vi "Write Array.vi"(8 "Error In":errorcluster, 10 "Name":string, 11 "Variant":variant) -> (0 "Error Out":errorcluster, 3 "String":string)   [LabVIEW 2017, in "Configit.lvlib"]
uses:
  Configit.lvlib
  <vilib>/Utility/VariantDataType/Type.ctl
  <vilib>/Waveform/DWDTOps.llb/DWDT Empty Digital.vi
  <vilib>/Waveform/DTblOps.llb/DTbl Empty Digital.vi
  <vilib>/Utility/VariantDataType/VariantType.lvlib
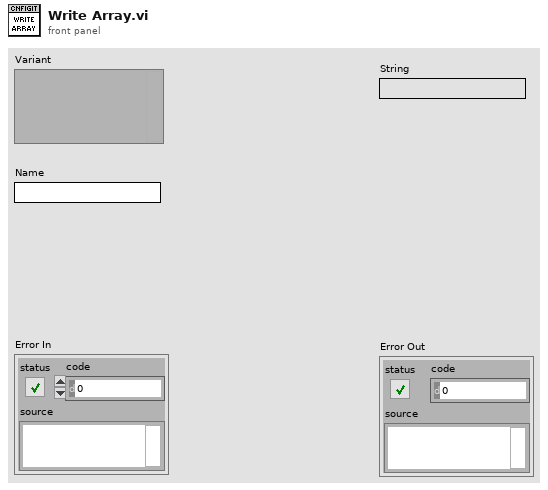
[diagram p1: front panel]
types:
  T1 = typedef "VariantType.lvlib/Type.ctl" = enum8{"Invalid Type", "Void", "I8", "I16", "I32", "I64", "U8", "U16", "U32", "U64", "Single Float", "Double Float", "Extended Float", "Single Complex", "Double Complex", "Extended Complex", "Enum U8", "Enum U16", "Enum U32", "Enum U64", "Single Float With Unit", "Double Float With Unit", "Extended Float With Unit", "Single Complex with Unit", "Double Complex with Unit", "Extended Complex with Unit", "Boolean", "String", "Path", "Picture", "Tag", "Array", "Cluster", "Variant", "LV Variant", "Waveform", "Timestamp", "Digital Waveform", "Digital Data", "ExpressData", "Refnum", "External Data", "VI", "Poly VI", "LabVIEW Class Instance", "Fixed Point"}
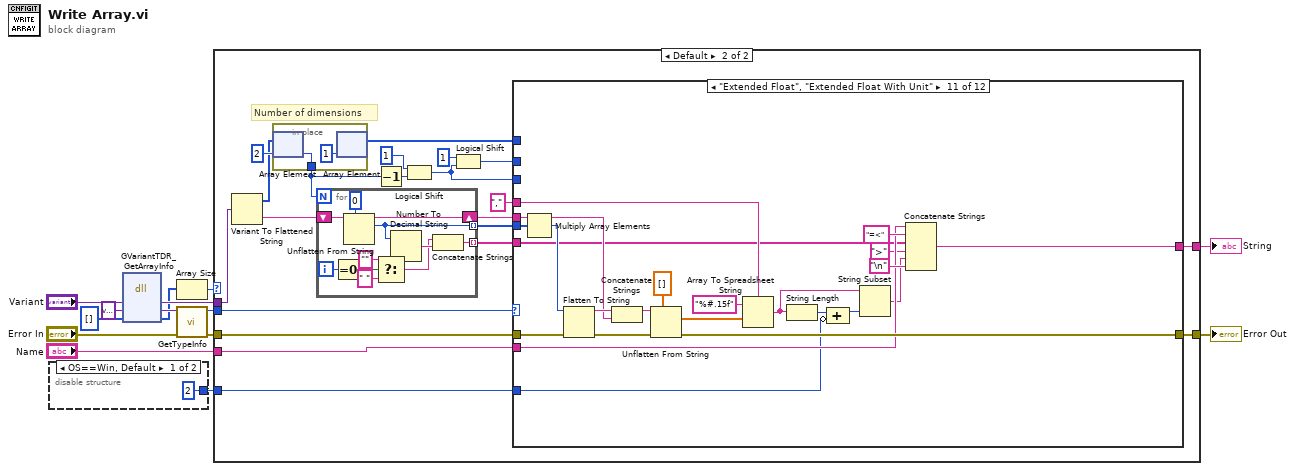
[diagram p0: block diagram]
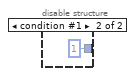
[diagram p2: hidden frame]
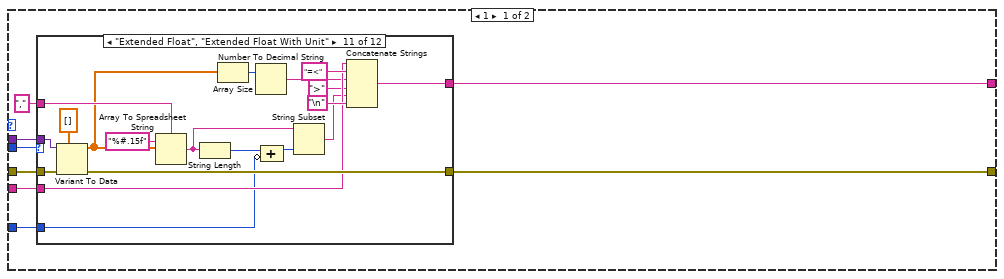
[diagram p3: hidden frame]
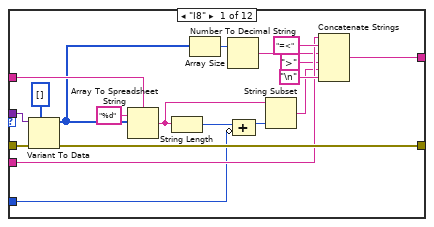
[diagram p4: hidden frame]
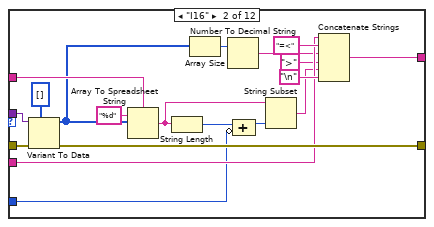
[diagram p5: hidden frame]
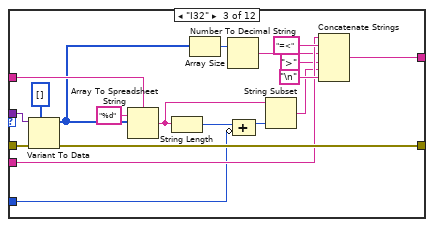
[diagram p6: hidden frame]
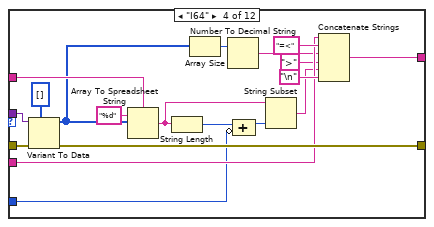
[diagram p7: hidden frame]
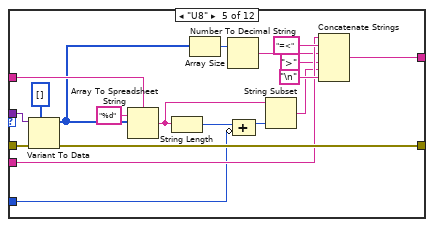
[diagram p8: hidden frame]
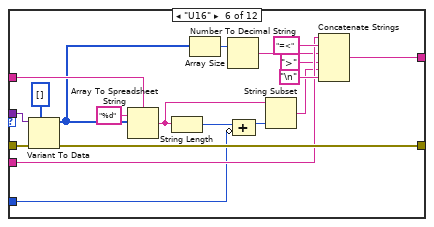
[diagram p9: hidden frame]
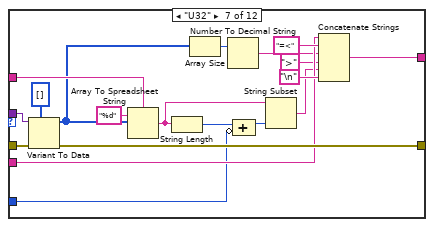
[diagram p10: hidden frame]
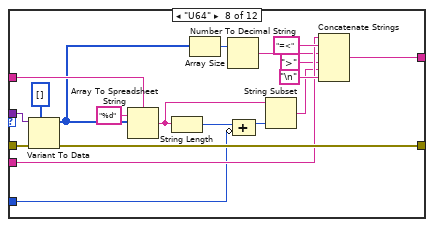
[diagram p11: hidden frame]
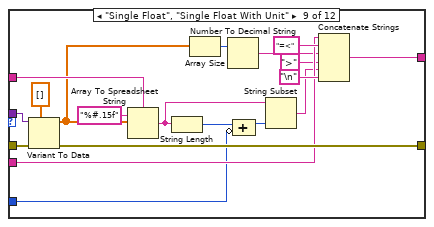
[diagram p12: hidden frame]
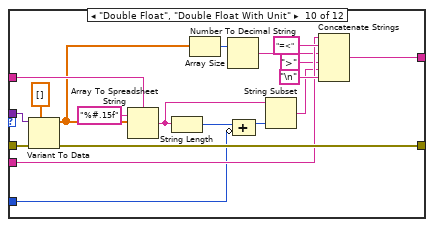
[diagram p13: hidden frame]
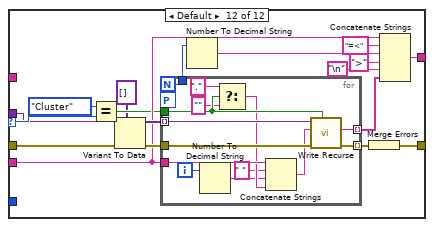
[diagram p14: hidden frame]
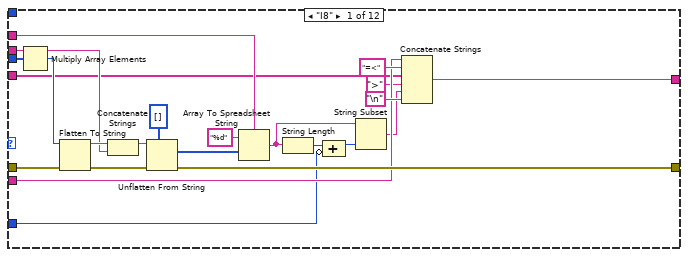
[diagram p15: hidden frame]
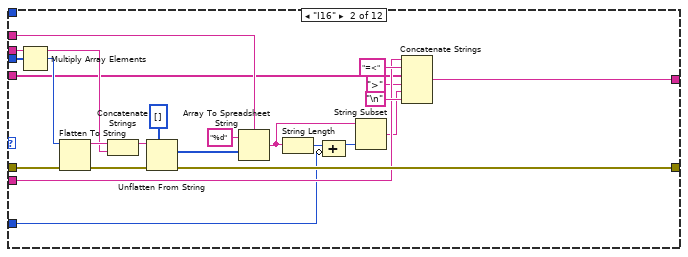
[diagram p16: hidden frame]
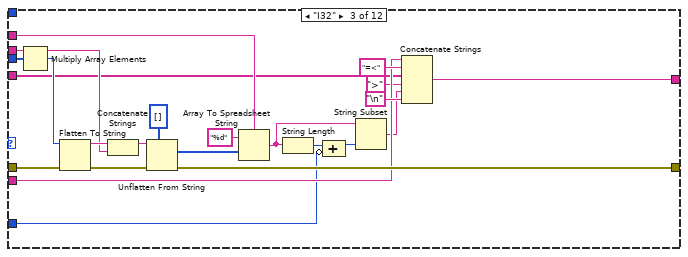
[diagram p17: hidden frame]
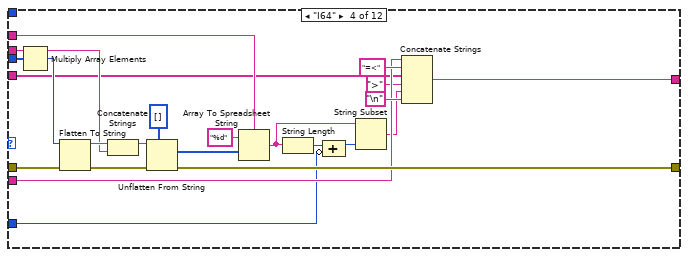
[diagram p18: hidden frame]
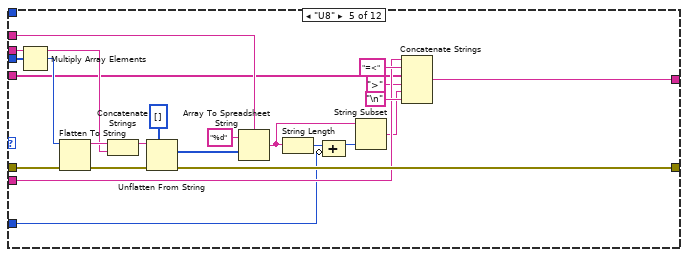
[diagram p19: hidden frame]
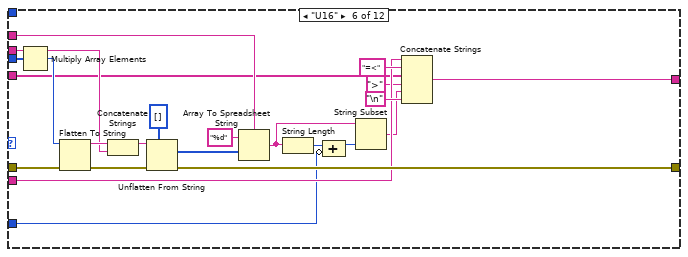
[diagram p20: hidden frame]
diagram:
  n1 = disable-structure shown="OS==Win, Default" {
    disable-tunnel: [2 ("value") 1 ("value")] -> w1
    frame condition #0 (active) {
    }
    frame condition #1 {
    }
  }
  n2 = dll-call lib="LabVIEW" fn="GVariantTDR_GetArrayInfo"("lvVar"="Variant", "eltType"=variant ("ArrayElt"), "dimInfo"=i32[] []) -> ("lvVar"=w4:variant, "eltType"=w6:variant, "dimInfo"=w3:i32[])  [unwired: 4 in, 2 out]
  n3 = Array Size(array=w3) -> (size(s)=w2:i32)
  n4 = call "GetTypeInfo.vi"("Error In"="Error In", "Variant"=w6) -> ("Error Out"=w13:errorcluster, "Type Enum"=w14:T1)  [unwired: 6 in, 2 out]
  n5 = case shown="Default" w2 {
    tunnel: w14 -> [w24 w284]
    tunnel: w13 -> [w23 w283]
    tunnel: [w21 w279] -> w12
    tunnel: [w20 w278] -> w11
    tunnel: "Name" -> [w19 w277]
    tunnel: w4 -> [w18 w276]
    tunnel: w1 -> [w17 w266]
    frame 1 {
      n6 = case shown="\"Extended Float\", \"Extended Float With Unit\"" w24 {
        selector: w24 -> [_ _ _ _ _ _ _ _ _ _ _ w246]
        tunnel: w23 -> [w34 w53 w72 w91 w110 w129 w148 w167 w186 w205 w224 w237]
        tunnel: "," -> [w41 w60 w79 w98 w117 w136 w155 w174 w193 w212 w231 _]
        tunnel: [w38 w57 w76 w95 w114 w133 w152 w171 w190 w209 w228 w248] -> w21
        tunnel: [w37 w56 w75 w94 w113 w132 w151 w170 w189 w208 w227 w247] -> w20
        tunnel: w19 -> [w36 w55 w74 w93 w112 w131 w150 w169 w188 w207 w226 w242]
        tunnel: w18 -> [w33 w52 w71 w90 w109 w128 w147 w166 w185 w204 w223 w236]
        tunnel: w17 -> [w25 w44 w63 w82 w101 w120 w139 w158 w177 w196 w215 _]
        frame "I8" {
          n7 = Variant To Data(error in=w34, type=i8[] [], Variant=w33) -> (data=w32:i8[], error out=w37:errorcluster)
          n8 = Array To Spreadsheet String(delimiter (Tab)=w41, array=w32, 3:"%d" ("format string")) -> (spreadsheet string=w27:string)
          n9 = String Length(string=w27) -> (length=w28:i32)
          n10 = Array Size(array=w32) -> (size(s)=w31:i32)
          n11 = Number To Decimal String(number=w31) -> (decimal integer string=w30:string)  [unwired: 1 in]
          n12 = Compound Arithmetic op=ADD(w28, invert w25) -> (w29:i32)
          n13 = String Subset(string=w27, length (rest)=w29) -> (substring=w26:string)  [unwired: 1 in]
          n14 = Concatenate Strings(w36, "=<" ("string"), w30, ">" ("string"), w26, "\n") -> (w38:string)
        }
        frame "I16" {
          n15 = Variant To Data(error in=w53, type=i16[] [], Variant=w52) -> (data=w51:i16[], error out=w56:errorcluster)
          n16 = Array To Spreadsheet String(delimiter (Tab)=w60, array=w51, 3:"%d" ("format string")) -> (spreadsheet string=w46:string)
          n17 = String Length(string=w46) -> (length=w47:i32)
          n18 = Array Size(array=w51) -> (size(s)=w50:i32)
          n19 = Number To Decimal String(number=w50) -> (decimal integer string=w49:string)  [unwired: 1 in]
          n20 = Compound Arithmetic op=ADD(w47, invert w44) -> (w48:i32)
          n21 = String Subset(string=w46, length (rest)=w48) -> (substring=w45:string)  [unwired: 1 in]
          n22 = Concatenate Strings(w55, "=<" ("string"), w49, ">" ("string"), w45, "\n") -> (w57:string)
        }
        frame "I32" {
          n23 = Variant To Data(error in=w72, type=i32[] [], Variant=w71) -> (data=w70:i32[], error out=w75:errorcluster)
          n24 = Array To Spreadsheet String(delimiter (Tab)=w79, array=w70, 3:"%d" ("format string")) -> (spreadsheet string=w65:string)
          n25 = String Length(string=w65) -> (length=w66:i32)
          n26 = Array Size(array=w70) -> (size(s)=w69:i32)
          n27 = Number To Decimal String(number=w69) -> (decimal integer string=w68:string)  [unwired: 1 in]
          n28 = Compound Arithmetic op=ADD(w66, invert w63) -> (w67:i32)
          n29 = String Subset(string=w65, length (rest)=w67) -> (substring=w64:string)  [unwired: 1 in]
          n30 = Concatenate Strings(w74, "=<" ("string"), w68, ">" ("string"), w64, "\n") -> (w76:string)
        }
        frame "I64" {
          n31 = Variant To Data(error in=w91, type=i64[] [], Variant=w90) -> (data=w89:i64[], error out=w94:errorcluster)
          n32 = Array To Spreadsheet String(delimiter (Tab)=w98, array=w89, 3:"%d" ("format string")) -> (spreadsheet string=w84:string)
          n33 = String Length(string=w84) -> (length=w85:i32)
          n34 = Array Size(array=w89) -> (size(s)=w88:i32)
          n35 = Number To Decimal String(number=w88) -> (decimal integer string=w87:string)  [unwired: 1 in]
          n36 = Compound Arithmetic op=ADD(w85, invert w82) -> (w86:i32)
          n37 = String Subset(string=w84, length (rest)=w86) -> (substring=w83:string)  [unwired: 1 in]
          n38 = Concatenate Strings(w93, "=<" ("string"), w87, ">" ("string"), w83, "\n") -> (w95:string)
        }
        frame "U8" {
          n39 = Variant To Data(error in=w110, type=u8[] [], Variant=w109) -> (data=w108:u8[], error out=w113:errorcluster)
          n40 = Array To Spreadsheet String(delimiter (Tab)=w117, array=w108, 3:"%d" ("format string")) -> (spreadsheet string=w103:string)
          n41 = String Length(string=w103) -> (length=w104:i32)
          n42 = Array Size(array=w108) -> (size(s)=w107:i32)
          n43 = Number To Decimal String(number=w107) -> (decimal integer string=w106:string)  [unwired: 1 in]
          n44 = Compound Arithmetic op=ADD(w104, invert w101) -> (w105:i32)
          n45 = String Subset(string=w103, length (rest)=w105) -> (substring=w102:string)  [unwired: 1 in]
          n46 = Concatenate Strings(w112, "=<" ("string"), w106, ">" ("string"), w102, "\n") -> (w114:string)
        }
        frame "U16" {
          n47 = Variant To Data(error in=w129, type=u16[] [], Variant=w128) -> (data=w127:u16[], error out=w132:errorcluster)
          n48 = Array To Spreadsheet String(delimiter (Tab)=w136, array=w127, 3:"%d" ("format string")) -> (spreadsheet string=w122:string)
          n49 = String Length(string=w122) -> (length=w123:i32)
          n50 = Array Size(array=w127) -> (size(s)=w126:i32)
          n51 = Number To Decimal String(number=w126) -> (decimal integer string=w125:string)  [unwired: 1 in]
          n52 = Compound Arithmetic op=ADD(w123, invert w120) -> (w124:i32)
          n53 = String Subset(string=w122, length (rest)=w124) -> (substring=w121:string)  [unwired: 1 in]
          n54 = Concatenate Strings(w131, "=<" ("string"), w125, ">" ("string"), w121, "\n") -> (w133:string)
        }
        frame "U32" {
          n55 = Variant To Data(error in=w148, type=u32[] [], Variant=w147) -> (data=w146:u32[], error out=w151:errorcluster)
          n56 = Array To Spreadsheet String(delimiter (Tab)=w155, array=w146, 3:"%d" ("format string")) -> (spreadsheet string=w141:string)
          n57 = String Length(string=w141) -> (length=w142:i32)
          n58 = Array Size(array=w146) -> (size(s)=w145:i32)
          n59 = Number To Decimal String(number=w145) -> (decimal integer string=w144:string)  [unwired: 1 in]
          n60 = Compound Arithmetic op=ADD(w142, invert w139) -> (w143:i32)
          n61 = String Subset(string=w141, length (rest)=w143) -> (substring=w140:string)  [unwired: 1 in]
          n62 = Concatenate Strings(w150, "=<" ("string"), w144, ">" ("string"), w140, "\n") -> (w152:string)
        }
        frame "U64" {
          n63 = Variant To Data(error in=w167, type=u64[] [], Variant=w166) -> (data=w165:u64[], error out=w170:errorcluster)
          n64 = Array To Spreadsheet String(delimiter (Tab)=w174, array=w165, 3:"%d" ("format string")) -> (spreadsheet string=w160:string)
          n65 = String Length(string=w160) -> (length=w161:i32)
          n66 = Array Size(array=w165) -> (size(s)=w164:i32)
          n67 = Number To Decimal String(number=w164) -> (decimal integer string=w163:string)  [unwired: 1 in]
          n68 = Compound Arithmetic op=ADD(w161, invert w158) -> (w162:i32)
          n69 = String Subset(string=w160, length (rest)=w162) -> (substring=w159:string)  [unwired: 1 in]
          n70 = Concatenate Strings(w169, "=<" ("string"), w163, ">" ("string"), w159, "\n") -> (w171:string)
        }
        frame "Single Float", "Single Float With Unit" {
          n71 = Variant To Data(error in=w186, type=sgl[] [], Variant=w185) -> (data=w184:sgl[], error out=w189:errorcluster)
          n72 = Array To Spreadsheet String(delimiter (Tab)=w193, array=w184, 3:"%#.15f" ("format string")) -> (spreadsheet string=w179:string)
          n73 = String Length(string=w179) -> (length=w180:i32)
          n74 = Array Size(array=w184) -> (size(s)=w183:i32)
          n75 = Number To Decimal String(number=w183) -> (decimal integer string=w182:string)  [unwired: 1 in]
          n76 = Compound Arithmetic op=ADD(w180, invert w177) -> (w181:i32)
          n77 = String Subset(string=w179, length (rest)=w181) -> (substring=w178:string)  [unwired: 1 in]
          n78 = Concatenate Strings(w188, "=<" ("string"), w182, ">" ("string"), w178, "\n") -> (w190:string)
        }
        frame "Double Float", "Double Float With Unit" {
          n79 = Variant To Data(error in=w205, type=dbl[] [], Variant=w204) -> (data=w203:dbl[], error out=w208:errorcluster)
          n80 = Array To Spreadsheet String(delimiter (Tab)=w212, array=w203, 3:"%#.15f" ("format string")) -> (spreadsheet string=w198:string)
          n81 = String Length(string=w198) -> (length=w199:i32)
          n82 = Array Size(array=w203) -> (size(s)=w202:i32)
          n83 = Number To Decimal String(number=w202) -> (decimal integer string=w201:string)  [unwired: 1 in]
          n84 = Compound Arithmetic op=ADD(w199, invert w196) -> (w200:i32)
          n85 = String Subset(string=w198, length (rest)=w200) -> (substring=w197:string)  [unwired: 1 in]
          n86 = Concatenate Strings(w207, "=<" ("string"), w201, ">" ("string"), w197, "\n") -> (w209:string)
        }
        frame "Extended Float", "Extended Float With Unit" {
          n87 = Variant To Data(error in=w224, type=ext[] [], Variant=w223) -> (data=w222:ext[], error out=w227:errorcluster)
          n88 = Array To Spreadsheet String(delimiter (Tab)=w231, array=w222, 3:"%#.15f" ("format string")) -> (spreadsheet string=w217:string)
          n89 = String Length(string=w217) -> (length=w218:i32)
          n90 = Array Size(array=w222) -> (size(s)=w221:i32)
          n91 = Number To Decimal String(number=w221) -> (decimal integer string=w220:string)  [unwired: 1 in]
          n92 = Compound Arithmetic op=ADD(w218, invert w215) -> (w219:i32)
          n93 = String Subset(string=w217, length (rest)=w219) -> (substring=w216:string)  [unwired: 1 in]
          n94 = Concatenate Strings(w226, "=<" ("string"), w220, ">" ("string"), w216, "\n") -> (w228:string)
        }
        frame Default {
          n95 = Equal?(x=Type."Cluster", y=w246) -> (x = y?=w241:bool)
          n96 = Variant To Data(error in=w237, type=variant[] [], Variant=w236) -> (data=w244:variant[], error out=w243:errorcluster)
          n97 = for {
            N -> [w255]
            tunnel: w244 -> [w263] mode=indexing
            tunnel: [w262] -> w239 mode=indexing
            tunnel: w242 -> [w261]
            tunnel: w241 -> [w259]
            workers-P: _ -> [_]
            tunnel: w243 -> [w265]
            tunnel: [w264] -> w240 mode=indexing
            tunnel: [w255] -> w235
            i -> [w252]
            n98 = Number To Decimal String(number=w252) -> (decimal integer string=w253:string)  [unwired: 1 in]
            n99 = Select(t="." ("string"), s=w259, f="") -> (s? t:f=w257:string)
            n100 = Concatenate Strings(w261, " " ("string"), w253, w257) -> (w260:string)
            n101 = call "Write Recurse.vi"("Append Name (T)"=w259, "Error In"=w265, "Name"=w260, "Variant"=w263) -> ("Error Out"=w264:errorcluster, "String"=w262:string)  [unwired: 6 in]
          }
          n102 = Number To Decimal String(number=w235) -> (decimal integer string=w234:string)  [unwired: 1 in]
          n103 = Merge Errors(w240) -> (w247:errorcluster)
          n104 = Concatenate Strings(w242, "=<" ("string"), w234, ">" ("string"), "\n", w239) -> (w248:string)
        }
      }
    }
    frame Default {
      # "Number of dimensions"
      n105 = Variant To Flattened String(Variant=w276) -> (data string=w286:string, 1:w274:i16[])
      n106 = in-place {
        in-place-border: [w287] -> w270
        n107 = in-place-array #1(w274, 2) -> (w287:i16)
        n108 = in-place-array #1(i16 1 ("element")) -> (w273:i16[])  [unwired: 1 out]
      }
      n109 = for {
        N: w270 -> [_]
        shift-right: [w615] -> w282
        shift-left: w286 -> [w616]
        tunnel: [w612] -> w285 mode=indexing
        tunnel: [w613] -> w280 mode=indexing
        i -> [w611]
        n110 = Equal To 0?(x=w611) -> (x = 0?=w610:bool)
        n111 = Unflatten From String(type=u32 0, binary string=w616) -> (rest of the binary string=w615:string, value=w612:u32)  [unwired: 3 in, 1 out]
        n112 = Select(t="", s=w610, f=" ") -> (s? t:f=w608:string)
        n113 = Number To Decimal String(number=w612) -> (decimal integer string=w614:string)  [unwired: 1 in]
        n114 = Concatenate Strings(w608, w614) -> (w613:string)
      }
      n115 = Decrement(x=w270) -> (x-1=w272:i16)
      n116 = Logical Shift(y=i16 1, x=w272) -> (x << y=w268:i16)
      n117 = Logical Shift(y=i16 1, x=w268) -> (x << y=w267:i16)
      n118 = case shown="\"Extended Float\", \"Extended Float With Unit\"" w284 {
        selector: w284 -> [_ _ _ _ _ _ _ _ _ _ _ w566]
        tunnel: w285 -> [w305 w328 w351 w374 w397 w420 w443 w466 w489 w512 w535 w555]
        tunnel: w283 -> [w306 w329 w352 w375 w398 w421 w444 w467 w490 w513 w536 w553]
        tunnel: w282 -> [w303 w326 w349 w372 w395 w418 w441 w464 w487 w510 w533 w554]
        tunnel: "," -> [w301 w324 w347 w370 w393 w416 w439 w462 w485 w508 w531 _]
        tunnel: w280 -> [w294 w317 w340 w363 w386 w409 w432 w455 w478 w501 w524 w569]
        tunnel: [w298 w321 w344 w367 w390 w413 w436 w459 w482 w505 w528 w568] -> w279
        tunnel: [w297 w320 w343 w366 w389 w412 w435 w458 w481 w504 w527 w567] -> w278
        tunnel: w277 -> [w296 w319 w342 w365 w388 w411 w434 w457 w480 w503 w526 w561]
        tunnel: w273 -> [_ _ _ _ _ _ _ _ _ _ _ w548]
        tunnel: w268 -> [_ _ _ _ _ _ _ _ _ _ _ w546]
        tunnel: w267 -> [_ _ _ _ _ _ _ _ _ _ _ w545]
        tunnel: w266 -> [w290 w313 w336 w359 w382 w405 w428 w451 w474 w497 w520 _]
        frame "I8" {
          n119 = Multiply Array Elements(1:w305) -> (0:w304:u32)
          n120 = Flatten To String(anything=w304, error in (no error)=w306) -> (data string=w309:string, error out=w311:errorcluster)  [unwired: 2 in, 1 out]
          n121 = Concatenate Strings(w309, w303) -> (w308:string)
          n122 = Unflatten From String(type=i8[] [], binary string=w308, error in (no error)=w311) -> (value=w310:i8[], error out=w297:errorcluster)  [unwired: 2 in, 1 out]
          n123 = Array To Spreadsheet String(delimiter (Tab)=w301, array=w310, 3:"%d" ("format string")) -> (spreadsheet string=w291:string)
          n124 = String Length(string=w291) -> (length=w292:i32)
          n125 = Compound Arithmetic op=ADD(w292, invert w290) -> (w293:i32)
          n126 = String Subset(string=w291, length (rest)=w293) -> (substring=w289:string)  [unwired: 1 in]
          n127 = Concatenate Strings(w296, "=<" ("string"), w294, ">" ("string"), w289, "\n") -> (w298:string)
        }
        frame "I16" {
          n128 = Multiply Array Elements(1:w328) -> (0:w327:u32)
          n129 = Flatten To String(anything=w327, error in (no error)=w329) -> (data string=w332:string, error out=w334:errorcluster)  [unwired: 2 in, 1 out]
          n130 = Concatenate Strings(w332, w326) -> (w331:string)
          n131 = Unflatten From String(type=i16[] [], binary string=w331, error in (no error)=w334) -> (value=w333:i16[], error out=w320:errorcluster)  [unwired: 2 in, 1 out]
          n132 = Array To Spreadsheet String(delimiter (Tab)=w324, array=w333, 3:"%d" ("format string")) -> (spreadsheet string=w314:string)
          n133 = String Length(string=w314) -> (length=w315:i32)
          n134 = Compound Arithmetic op=ADD(w315, invert w313) -> (w316:i32)
          n135 = String Subset(string=w314, length (rest)=w316) -> (substring=w312:string)  [unwired: 1 in]
          n136 = Concatenate Strings(w319, "=<" ("string"), w317, ">" ("string"), w312, "\n") -> (w321:string)
        }
        frame "I32" {
          n137 = Multiply Array Elements(1:w351) -> (0:w350:u32)
          n138 = Flatten To String(anything=w350, error in (no error)=w352) -> (data string=w355:string, error out=w357:errorcluster)  [unwired: 2 in, 1 out]
          n139 = Concatenate Strings(w355, w349) -> (w354:string)
          n140 = Unflatten From String(type=i32[] [], binary string=w354, error in (no error)=w357) -> (value=w356:i32[], error out=w343:errorcluster)  [unwired: 2 in, 1 out]
          n141 = Array To Spreadsheet String(delimiter (Tab)=w347, array=w356, 3:"%d" ("format string")) -> (spreadsheet string=w337:string)
          n142 = String Length(string=w337) -> (length=w338:i32)
          n143 = Compound Arithmetic op=ADD(w338, invert w336) -> (w339:i32)
          n144 = String Subset(string=w337, length (rest)=w339) -> (substring=w335:string)  [unwired: 1 in]
          n145 = Concatenate Strings(w342, "=<" ("string"), w340, ">" ("string"), w335, "\n") -> (w344:string)
        }
        frame "I64" {
          n146 = Multiply Array Elements(1:w374) -> (0:w373:u32)
          n147 = Flatten To String(anything=w373, error in (no error)=w375) -> (data string=w378:string, error out=w380:errorcluster)  [unwired: 2 in, 1 out]
          n148 = Concatenate Strings(w378, w372) -> (w377:string)
          n149 = Unflatten From String(type=i64[] [], binary string=w377, error in (no error)=w380) -> (value=w379:i64[], error out=w366:errorcluster)  [unwired: 2 in, 1 out]
          n150 = Array To Spreadsheet String(delimiter (Tab)=w370, array=w379, 3:"%d" ("format string")) -> (spreadsheet string=w360:string)
          n151 = String Length(string=w360) -> (length=w361:i32)
          n152 = Compound Arithmetic op=ADD(w361, invert w359) -> (w362:i32)
          n153 = String Subset(string=w360, length (rest)=w362) -> (substring=w358:string)  [unwired: 1 in]
          n154 = Concatenate Strings(w365, "=<" ("string"), w363, ">" ("string"), w358, "\n") -> (w367:string)
        }
        frame "U8" {
          n155 = Multiply Array Elements(1:w397) -> (0:w396:u32)
          n156 = Flatten To String(anything=w396, error in (no error)=w398) -> (data string=w401:string, error out=w403:errorcluster)  [unwired: 2 in, 1 out]
          n157 = Concatenate Strings(w401, w395) -> (w400:string)
          n158 = Unflatten From String(type=u8[] [], binary string=w400, error in (no error)=w403) -> (value=w402:u8[], error out=w389:errorcluster)  [unwired: 2 in, 1 out]
          n159 = Array To Spreadsheet String(delimiter (Tab)=w393, array=w402, 3:"%d" ("format string")) -> (spreadsheet string=w383:string)
          n160 = String Length(string=w383) -> (length=w384:i32)
          n161 = Compound Arithmetic op=ADD(w384, invert w382) -> (w385:i32)
          n162 = String Subset(string=w383, length (rest)=w385) -> (substring=w381:string)  [unwired: 1 in]
          n163 = Concatenate Strings(w388, "=<" ("string"), w386, ">" ("string"), w381, "\n") -> (w390:string)
        }
        frame "U16" {
          n164 = Multiply Array Elements(1:w420) -> (0:w419:u32)
          n165 = Flatten To String(anything=w419, error in (no error)=w421) -> (data string=w424:string, error out=w426:errorcluster)  [unwired: 2 in, 1 out]
          n166 = Concatenate Strings(w424, w418) -> (w423:string)
          n167 = Unflatten From String(type=u16[] [], binary string=w423, error in (no error)=w426) -> (value=w425:u16[], error out=w412:errorcluster)  [unwired: 2 in, 1 out]
          n168 = Array To Spreadsheet String(delimiter (Tab)=w416, array=w425, 3:"%d" ("format string")) -> (spreadsheet string=w406:string)
          n169 = String Length(string=w406) -> (length=w407:i32)
          n170 = Compound Arithmetic op=ADD(w407, invert w405) -> (w408:i32)
          n171 = String Subset(string=w406, length (rest)=w408) -> (substring=w404:string)  [unwired: 1 in]
          n172 = Concatenate Strings(w411, "=<" ("string"), w409, ">" ("string"), w404, "\n") -> (w413:string)
        }
        frame "U32" {
          n173 = Multiply Array Elements(1:w443) -> (0:w442:u32)
          n174 = Flatten To String(anything=w442, error in (no error)=w444) -> (data string=w447:string, error out=w449:errorcluster)  [unwired: 2 in, 1 out]
          n175 = Concatenate Strings(w447, w441) -> (w446:string)
          n176 = Unflatten From String(type=u32[] [], binary string=w446, error in (no error)=w449) -> (value=w448:u32[], error out=w435:errorcluster)  [unwired: 2 in, 1 out]
          n177 = Array To Spreadsheet String(delimiter (Tab)=w439, array=w448, 3:"%d" ("format string")) -> (spreadsheet string=w429:string)
          n178 = String Length(string=w429) -> (length=w430:i32)
          n179 = Compound Arithmetic op=ADD(w430, invert w428) -> (w431:i32)
          n180 = String Subset(string=w429, length (rest)=w431) -> (substring=w427:string)  [unwired: 1 in]
          n181 = Concatenate Strings(w434, "=<" ("string"), w432, ">" ("string"), w427, "\n") -> (w436:string)
        }
        frame "U64" {
          n182 = Multiply Array Elements(1:w466) -> (0:w465:u32)
          n183 = Flatten To String(anything=w465, error in (no error)=w467) -> (data string=w470:string, error out=w472:errorcluster)  [unwired: 2 in, 1 out]
          n184 = Concatenate Strings(w470, w464) -> (w469:string)
          n185 = Unflatten From String(type=u64[] [], binary string=w469, error in (no error)=w472) -> (value=w471:u64[], error out=w458:errorcluster)  [unwired: 2 in, 1 out]
          n186 = Array To Spreadsheet String(delimiter (Tab)=w462, array=w471, 3:"%d" ("format string")) -> (spreadsheet string=w452:string)
          n187 = String Length(string=w452) -> (length=w453:i32)
          n188 = Compound Arithmetic op=ADD(w453, invert w451) -> (w454:i32)
          n189 = String Subset(string=w452, length (rest)=w454) -> (substring=w450:string)  [unwired: 1 in]
          n190 = Concatenate Strings(w457, "=<" ("string"), w455, ">" ("string"), w450, "\n") -> (w459:string)
        }
        frame "Single Float", "Single Float With Unit" {
          n191 = Multiply Array Elements(1:w489) -> (0:w488:u32)
          n192 = Flatten To String(anything=w488, error in (no error)=w490) -> (data string=w493:string, error out=w495:errorcluster)  [unwired: 2 in, 1 out]
          n193 = Concatenate Strings(w493, w487) -> (w492:string)
          n194 = Unflatten From String(type=sgl[] [], binary string=w492, error in (no error)=w495) -> (value=w494:sgl[], error out=w481:errorcluster)  [unwired: 2 in, 1 out]
          n195 = Array To Spreadsheet String(delimiter (Tab)=w485, array=w494, 3:"%#.15f" ("format string")) -> (spreadsheet string=w475:string)
          n196 = String Length(string=w475) -> (length=w476:i32)
          n197 = Compound Arithmetic op=ADD(w476, invert w474) -> (w477:i32)
          n198 = String Subset(string=w475, length (rest)=w477) -> (substring=w473:string)  [unwired: 1 in]
          n199 = Concatenate Strings(w480, "=<" ("string"), w478, ">" ("string"), w473, "\n") -> (w482:string)
        }
        frame "Double Float", "Double Float With Unit" {
          n200 = Multiply Array Elements(1:w512) -> (0:w511:u32)
          n201 = Flatten To String(anything=w511, error in (no error)=w513) -> (data string=w516:string, error out=w518:errorcluster)  [unwired: 2 in, 1 out]
          n202 = Concatenate Strings(w516, w510) -> (w515:string)
          n203 = Unflatten From String(type=dbl[] [], binary string=w515, error in (no error)=w518) -> (value=w517:dbl[], error out=w504:errorcluster)  [unwired: 2 in, 1 out]
          n204 = Array To Spreadsheet String(delimiter (Tab)=w508, array=w517, 3:"%#.15f" ("format string")) -> (spreadsheet string=w498:string)
          n205 = String Length(string=w498) -> (length=w499:i32)
          n206 = Compound Arithmetic op=ADD(w499, invert w497) -> (w500:i32)
          n207 = String Subset(string=w498, length (rest)=w500) -> (substring=w496:string)  [unwired: 1 in]
          n208 = Concatenate Strings(w503, "=<" ("string"), w501, ">" ("string"), w496, "\n") -> (w505:string)
        }
        frame "Extended Float", "Extended Float With Unit" {
          n209 = Multiply Array Elements(1:w535) -> (0:w534:u32)
          n210 = Flatten To String(anything=w534, error in (no error)=w536) -> (data string=w539:string, error out=w541:errorcluster)  [unwired: 2 in, 1 out]
          n211 = Concatenate Strings(w539, w533) -> (w538:string)
          n212 = Unflatten From String(type=ext[] [], binary string=w538, error in (no error)=w541) -> (value=w540:ext[], error out=w527:errorcluster)  [unwired: 2 in, 1 out]
          n213 = Array To Spreadsheet String(delimiter (Tab)=w531, array=w540, 3:"%#.15f" ("format string")) -> (spreadsheet string=w521:string)
          n214 = String Length(string=w521) -> (length=w522:i32)
          n215 = Compound Arithmetic op=ADD(w522, invert w520) -> (w523:i32)
          n216 = String Subset(string=w521, length (rest)=w523) -> (substring=w519:string)  [unwired: 1 in]
          n217 = Concatenate Strings(w526, "=<" ("string"), w524, ">" ("string"), w519, "\n") -> (w528:string)
        }
        frame Default {
          # "remove dimension lengths"
          # "length"
          n218 = Multiply Array Elements(1:w555) -> (0:w556:u32)
          n219 = Reverse 1D Array(array=w555) -> (reversed array=w573:u32[])
          n220 = in-place {
            in-place-border: w545 -> [w579]
            n221 = in-place-array #2(w548, 0) -> (w581:i16)
            n222 = Compound Arithmetic op=ADD(w581, invert w579) -> (w580:i16)
            n223 = in-place-array #2(w580) -> (w550:i16[])  [unwired: 1 out]
          }
          n224 = Flatten To String(anything=w556) -> (data string=w557:string)  [unwired: 3 in, 2 out]
          n225 = Delete From Array(array=w573) -> (array with subset deleted=w574:u32[])  [unwired: 2 in, 1 out]
          n226 = Equal?(x=Type."Cluster", y=w566) -> (x = y?=w560:bool)
          n227 = Concatenate Strings(w557, w554) -> (w552:string)
          n228 = for {
            tunnel: w574 -> [w606] mode=indexing
            tunnel: [w604] -> w576 mode=indexing
            border: u32 1 -> [_]
            n229 = feedback #3() -> (w605:u32)
            n230 = Compound Arithmetic op=MULTIPLY(w605, w606) -> (w604:u32)
            n231 = feedback-in #3(w604) -> ()
          }
          n232 = Delete From Array(array=w550, length=w546, index=3) -> (array with subset deleted=w547:i16[])  [unwired: 1 out]
          n233 = Reverse 1D Array(array=w576) -> (reversed array=w577:u32[])
          n234 = Flattened String To Variant(4:w553, 6:w552, 7:w547) -> (0:w543:errorcluster, 3:w542:variant)
          n235 = Variant To Data(error in=w543, type=variant[] [], Variant=w542) -> (data=w564:variant[], error out=w563:errorcluster)
          n236 = Build Array (concatenate)(w577, u32 1) -> (w562:u32[])
          n237 = for {
            N -> [w587]
            tunnel: w564 -> [w593] mode=indexing
            tunnel: [w592] -> w558 mode=indexing
            tunnel: w561 -> [w591]
            tunnel: w562 -> [w588]
            tunnel: w560 -> [w585]
            workers-P: _ -> [_]
            tunnel: w563 -> [w595]
            tunnel: [w594] -> w559 mode=indexing
            i -> [w589]
            n238 = for {
              tunnel: [w602] -> w586 mode=indexing
              tunnel: w589 -> [w600]
              tunnel: w588 -> [w596] mode=indexing
              shift-right: [w596] -> _
              shift-left: w587 -> [w597]
              n239 = Quotient & Remainder(x=w600, y=w597) -> (x-y*floor(x/y)=w601:u32)  [unwired: 1 out]
              n240 = Quotient & Remainder(x=w601, y=w596) -> (floor(x/y)=w599:u32)  [unwired: 1 out]
              n241 = Number To Decimal String(number=w599) -> (decimal integer string=w603:string)  [unwired: 1 in]
              n242 = Concatenate Strings(" " ("string"), w603) -> (w602:string)
            }
            n243 = Select(t="." ("string"), s=w585, f="") -> (s? t:f=w583:string)
            n244 = Concatenate Strings(w591, w586, w583) -> (w590:string)
            n245 = call "Write Recurse.vi"("Append Name (T)"=w585, "Error In"=w595, "Name"=w590, "Variant"=w593) -> ("Error Out"=w594:errorcluster, "String"=w592:string)  [unwired: 6 in]
          }
          n246 = Merge Errors(w559) -> (w567:errorcluster)
          n247 = Concatenate Strings(w561, "=<" ("string"), w569, ">" ("string"), "\n", w558) -> (w568:string)
        }
      }
    }
  }
  "Error Out" <- w11
  "String" <- w12
